vi "Read phase.vi"(8 "error in (no error)":errorcluster, 11 "VISA resource name":refnum<visa-resource-name>) -> (0 "error out":errorcluster, 1 "phase":dbl, 3 "VISA resource name out":refnum<visa-resource-name>)   [LabVIEW 2009, in "SR830.lvlib"]
doc: "Reads the phase of the lock-in amplifier."
uses:
  sr830/SR830.lvlib
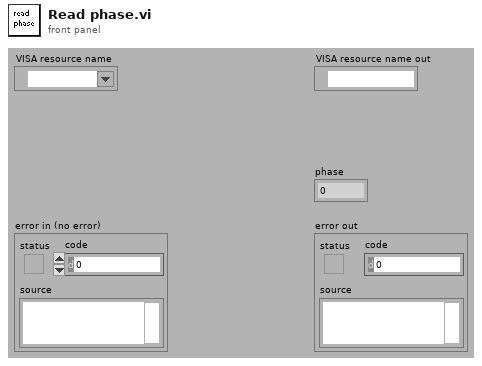
[diagram p1: front panel]
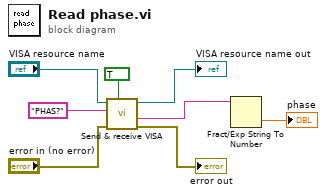
[diagram p0: block diagram]
diagram:
  n1 = call "Send & receive VISA.vi"("read? (f)"=TRUE, "error in (no error)"="error in (no error)", "write buffer"="PHAS?", "VISA resource name"="VISA resource name") -> ("error out"=→"error out":errorcluster, "read buffer"=w2:string, "VISA resource name out"=→"VISA resource name out":refnum<visa-resource-name>)  [unwired: 1 in, 4 out]
  n2 = Fract/Exp String To Number(string=w2) -> (number=→"phase":dbl)  [unwired: 4 out]
